vi "_QueueNames.vi"(8 "error in (no error)":errorcluster, 11 "MDPtrMgr in":refnum<class "MDPtrMgr.lvclass">) -> (0 "error out":errorcluster, 2 "Queue Names":string[](array[string]), 3 "MDPtrMgr out":refnum<class "MDPtrMgr.lvclass">)   [LabVIEW 2017, in "MDPtr.lvlib" / "MDPtrMgr.lvclass"]
uses:
  MDPtrMgr.lvclass
  MDPtrMgr.lvclass/MDPtrMgr.ctl
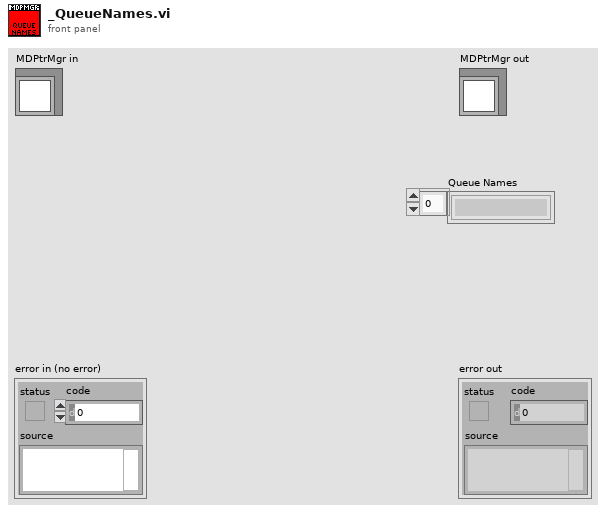
[diagram p1: front panel]
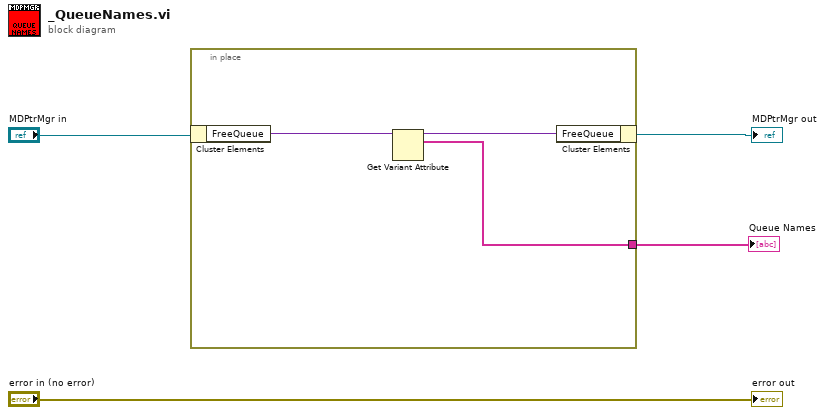
[diagram p0: block diagram]
diagram:
  n1 = in-place {
    in-place-border: [w5] -> w1
    n2 = in-place-cluster #1("MDPtrMgr in") -> ("FreeQueue"=w7:variant)
    n3 = Get Variant Attribute(Variant=w7) -> (duplicate Variant=w6:variant, names=w5:string[])  [unwired: 3 in, 2 out]
    n4 = in-place-cluster #1("FreeQueue"=w6) -> (→"MDPtrMgr out":refnum<class "MDPtrMgr.lvclass">)
  }
  "Queue Names" <- w1
  "error out" <- "error in (no error)"
